vi "get_weights.vi"(8 "Output Size":i32, 9 "2H Size":i32, 10 "1H Size":i32, 11 "Input Size":i32) -> (3 "Weights & Biases":T1)   [LabVIEW 2018]
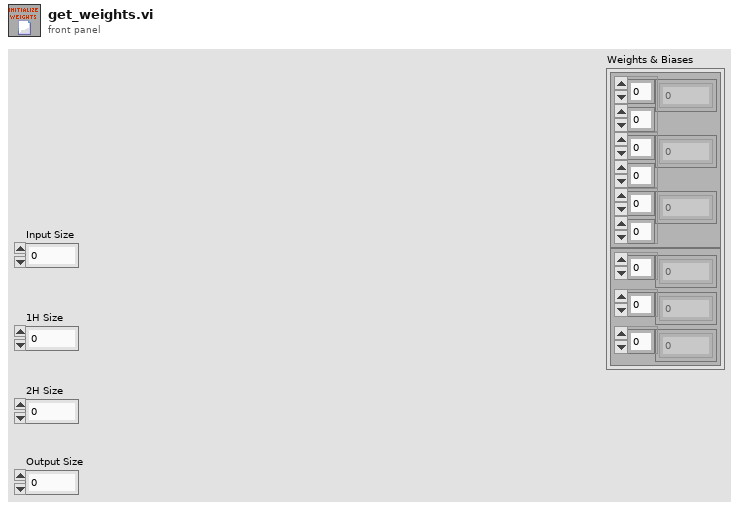
[diagram p1: front panel]
types:
  T1 = cluster{cluster{dbl[][], dbl[][], dbl[][]}, cluster{dbl[], dbl[], dbl[]}}
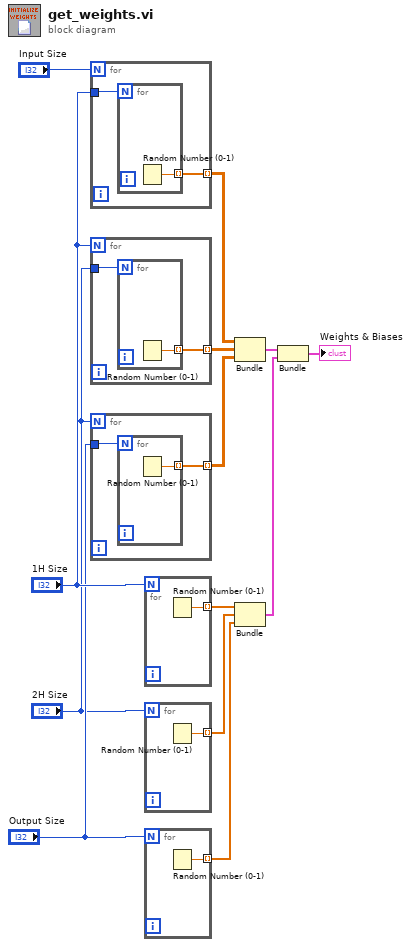
[diagram p0: block diagram]
diagram:
  n1 = for {
    N: "Input Size" -> [_]
    tunnel: [w15] -> w13 mode=indexing
    tunnel: "1H Size" -> [w14]
    n2 = for {
      N: w14 -> [_]
      tunnel: [w16] -> w15 mode=indexing
      n3 = Random Number (0-1)() -> (number: 0 to 1=w16:dbl)
    }
  }
  n4 = for {
    N: "1H Size" -> [_]
    tunnel: [w18] -> w12 mode=indexing
    tunnel: "2H Size" -> [w17]
    n5 = for {
      N: w17 -> [_]
      tunnel: [w19] -> w18 mode=indexing
      n6 = Random Number (0-1)() -> (number: 0 to 1=w19:dbl)
    }
  }
  n7 = for {
    N: "2H Size" -> [_]
    tunnel: [w21] -> w11 mode=indexing
    tunnel: "Output Size" -> [w20]
    n8 = for {
      N: w20 -> [_]
      tunnel: [w22] -> w21 mode=indexing
      n9 = Random Number (0-1)() -> (number: 0 to 1=w22:dbl)
    }
  }
  n10 = for {
    N: "1H Size" -> [_]
    tunnel: [w23] -> w10 mode=indexing
    n11 = Random Number (0-1)() -> (number: 0 to 1=w23:dbl)
  }
  n12 = for {
    N: "2H Size" -> [_]
    tunnel: [w24] -> w9 mode=indexing
    n13 = Random Number (0-1)() -> (number: 0 to 1=w24:dbl)
  }
  n14 = for {
    N: "Output Size" -> [_]
    tunnel: [w25] -> w8 mode=indexing
    n15 = Random Number (0-1)() -> (number: 0 to 1=w25:dbl)
  }
  n16 = Bundle(w13, w12, w11) -> (w3:cluster{dbl[][], dbl[][], dbl[][]})  [unwired: 1 in]
  n17 = Bundle(w10, w9, w8) -> (w2:cluster{dbl[], dbl[], dbl[]})  [unwired: 1 in]
  n18 = Bundle(w3, w2) -> (→"Weights & Biases":T1)  [unwired: 1 in]
